vi "StartSubroutine.vi"(8 "error in (no error)":errorcluster, 11 "AutoDrive in":refnum<class "AutoDrive.lvclass">) -> (0 "error out":errorcluster, 3 "AutoDrive out":refnum<class "AutoDrive.lvclass">)   [LabVIEW 2017]
uses:
  DriveAuto.lvclass
  AutoSubsystem/AutoSubroutine.lvclass
  AutoSubsystem/AutoDrive/AutoDrive.lvclass
panel:
  # "Re-Zero the gyro"
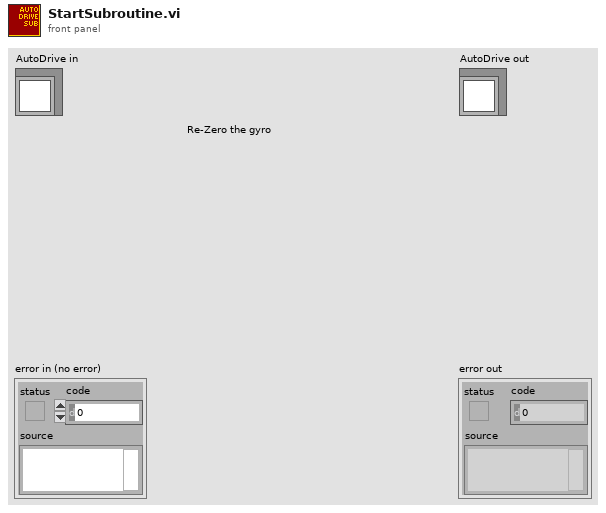
[diagram p1: front panel]
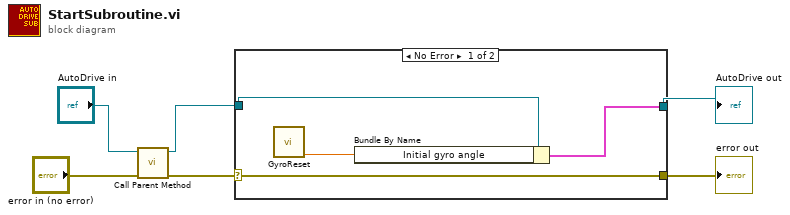
[diagram p0: block diagram]
diagram:
  n1 = call-parent "Call Parent Method"("error in (no error)"="error in (no error)", "AutoSubroutine in"="AutoDrive in") -> ("error out"=w4:errorcluster, "AutoSubroutine out"=w2:refnum<class "AutoSubroutine.lvclass">)  [unwired: 8 in]
  n2 = case shown="No Error" w4 {
    selector: w4 -> [w10 w11]
    tunnel: [w10 w11] -> w3
    tunnel: [w8 w12] -> w1
    tunnel: w2 -> [w9 w12]
    frame No Error {
      n3 = call "GyroReset.vi"() -> ("Heading"=w7:dbl)  [unwired: 11 in]
      n4 = Bundle By Name(cluster=w9, "Initial gyro angle"=w7) -> (w8:cluster{})
    }
    frame Error {
    }
  }
  "error out" <- w3
  "AutoDrive out" <- w1
